vi "Measure.vi"(6 "error in (no error)":errorcluster, 8 "Array of Measurement to Write":dbl[](array[numeric]), 9 "Generic Instrument in":refnum<class "Generic Instrument.lvclass">) -> (0 "error out":errorcluster, 2 "Array of Measurement":dbl[](array[numeric]), 3 "Generic Instrument out":refnum<class "Generic Instrument.lvclass">)   [LabVIEW 2013, in "Generic Instrument.lvlib" / "Generic Instrument.lvclass"]
uses:
  Generic Instrument.lvclass
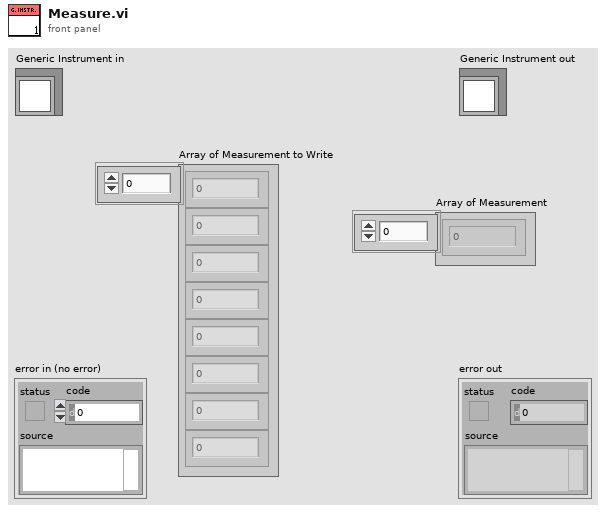
[diagram p1: front panel]
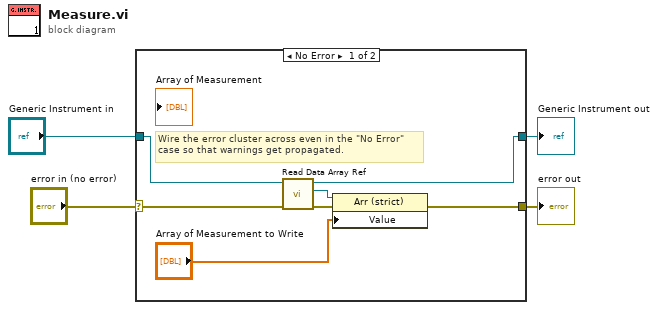
[diagram p0: block diagram]
diagram:
  n1 = case shown="No Error" "error in (no error)" {
    selector: "error in (no error)" -> [w6 w13]
    tunnel: [w8 w13] -> w3
    tunnel: [w11 w12] -> w1
    tunnel: "Generic Instrument in" -> [w7 w12]
    frame No Error {
      # "Wire the error cluster across even in the \"No Error\"\ncase so that warnings get propagated."
      n2 = call-dynamic "Read Data Array Ref.vi"("error in (no error)"=w6, "Generic Instrument in"=w7) -> ("error out"=w9:errorcluster, "Data Array Ref"=w10:refnum<vi>, "Generic Instrument out"=w11:refnum<class "Generic Instrument.lvclass">)  [unwired: 7 in]
      n3 = property class="Arr (strict)"(reference=w10, error in=w9, "Value"="Array of Measurement to Write") -> (error out=w8:errorcluster)  [unwired: 1 out]
    }
    frame Error {
    }
  }
  "error out" <- w3
  "Generic Instrument out" <- w1
